vi "K Calculation.vi"(11 "k_lqr":dbl) -> ()   [LabVIEW 2016]
uses:
  Globale Variable/Globale Variable.vi
  <vilib>/imath/engines/lvmath/Plug In/Control Design/BuiltInFunctions/lqr/NIMS_CD_lqr(A,B,Q,R,N).vi
  <vilib>/imath/engines/lvmath2/RunTimeEngine/NodeEndStatement/NIMS_NodeEndStatement_Get Scalar.vi
  <instcachedir>/0/NIMS_NodeEndStatement_Get Scalar_97655AD11A604E71BB6022AEBD8FDCD7.lvgen/NIMS_NodeEndStatement_Get Scalar_97655AD11A604E71BB6022AEBD8FDCD7_000.vi
  <vilib>/imath/engines/lvmath/Functions/Error Handling/MergeErrorsWrapper.vi
  <vilib>/imath/engines/lvmath2/RunTimeEngine/NodeEndStatement/NIMS_NodeEndStatement_Output.vi
  <instcachedir>/0/NIMS_NodeEndStatement_Output_53EC0D466D134D7ABD903AC30B43404B.lvgen/NIMS_NodeEndStatement_Output_53EC0D466D134D7ABD903AC30B43404B_001.vi
  <vilib>/imath/engines/lvmath2/RunTimeEngine/ErrorHandling/NIMS_Finalize Error.vi
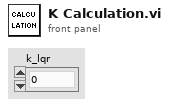
[diagram p1: front panel]
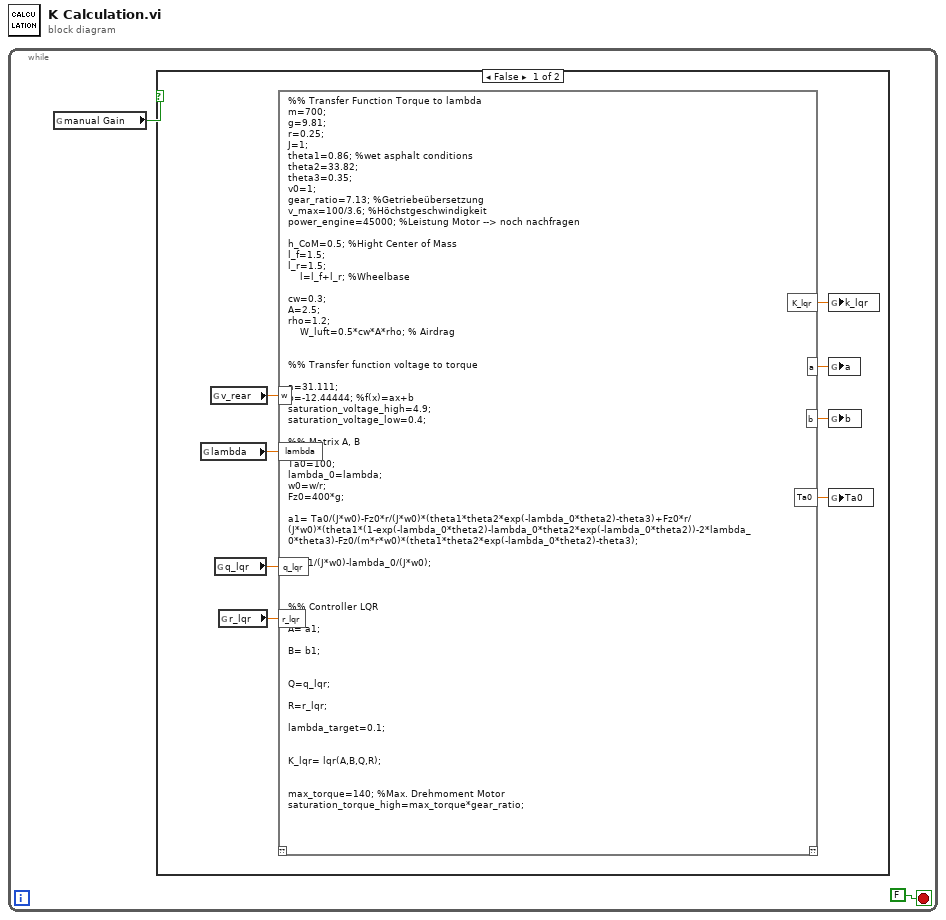
[diagram p0: block diagram]
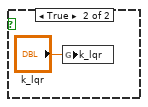
[diagram p2: hidden frame]
diagram:
  n1 = while {
    stop <- FALSE stop-if-true
    n2 = global read "Globale Variable.vi" "manual Gain"() -> (w2:bool)
    n3 = case shown="False" w2 {
      frame False {
        n4 = global read "Globale Variable.vi" "lambda"() -> (w8:dbl)
        n5 = global read "Globale Variable.vi" "v_rear"() -> (w9:dbl)
        n6 = global read "Globale Variable.vi" "q_lqr"() -> (w7:dbl)
        n7 = global read "Globale Variable.vi" "r_lqr"() -> (w6:dbl)
        n8 = mathscript code="%% Transfer Function Torque to lambda\nm=700;\ng=9.81;\nr=0.25;\nJ=1;\ntheta1=0.86; %wet asphalt conditions\ntheta2=33.82;\ntheta3=0.35;\nv0=1;\ngear_ratio=7.13; %Getriebeübersetzung\nv_max=100/3.6; %Höchstgeschwindigkeit\npower_engine=45000; %Leistung Motor --> noch nachfragen\n\nh_CoM=0.5; %Hight Center of Mass\nl_f=1.5; \nl_r=1.5;\n    l=l_f+l_r; %Wheelbase\n    \ncw=0.3;\nA=2.5;\nrho=1.2;\n    W_luft=0.5*cw*A*rho; % Airdrag\n    \n\n%% Transfer function voltage to torque\n\na=31.111;\nb=-12.44444; %f(x)=ax+b\nsaturation_voltage_high=4.9;\nsaturation_voltage_low=0.4;\n\n%% Matrix A, B\n\nTa0=100;\nlambda_0=lambda;\nw0=w/r;\nFz0=400*g;\n\na1= Ta0/(J*w0)-Fz0*r/(J*w0)*(theta1*theta2*exp(-lambda_0*theta2)-theta3)+Fz0*r/(J*w0)*(theta1*(1-exp(-lambda_0*theta2)-lambda_0*theta2*exp(-lambda_0*theta2))-2*lambda_0*theta3)-Fz0/(m*r*w0)*(theta1*theta2*exp(-lambda_0*theta2)-theta3);\n\nb1=1/(J*w0)-lambda_0/(J*w0);\n\n\n\n%% Controller LQR\n\nA= a1;\n\nB= b1;\n\n\nQ=q_lqr;\n\nR=r_lqr;\n\nlambda_target=0.1;\n\n\nK_lqr= lqr(A,B,Q,R);\n\n \nmax_torque=140; %Max. Drehmoment Motor\nsaturation_torque_high=max_torque*gear_ratio;"("w"=w9, "lambda"=w8, "q_lqr"=w7, "r_lqr"=w6) -> ("K_lqr"=w10:dbl, "a"=w5:dbl, "b"=w4:dbl, "Ta0"=w3:dbl)  [unwired: 1 in, 1 out]
        n9 = global write "Globale Variable.vi" "k_lqr"(w10) -> ()
        n10 = global write "Globale Variable.vi" "a"(w5) -> ()
        n11 = global write "Globale Variable.vi" "b"(w4) -> ()
        n12 = global write "Globale Variable.vi" "Ta0"(w3) -> ()
      }
      frame True {
        n13 = global write "Globale Variable.vi" "k_lqr"("k_lqr") -> ()
      }
    }
  }
